vi "Subtract XY (single).vi"(8 "error in (no error)":errorcluster, 9 "y":cluster{"X-array":dbl[], "Y-array":dbl[]}, 10 "x":cluster{"X-array":dbl[], "Y-array":dbl[]}, 11 "XY-data":cluster{"X-array":dbl[], "Y-array":dbl[]}) -> (0 "error out":errorcluster, 3 "XY-data out":cluster{"X-array":dbl[], "Y-array":dbl[]} {"Y-array" format="%.2p"; "X-array" format="%.2p"})   [LabVIEW 2016, in "xy_utilities.lvlib"]
doc: "Computes the difference of the inputs.\n\n<b>x</b>'s x array is subtracted from the x array of <b>XY-data</b>\n<b>y</b>'s y array is subtracted from the y array of <b>XY-data</b>\n\nWire data to the data input to determine the polymorphic instance to use or manually select the instance."
uses:
  xy_utilities.lvlib
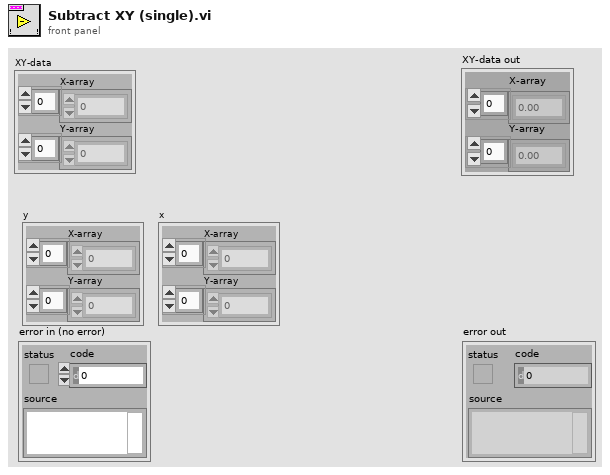
[diagram p1: front panel]
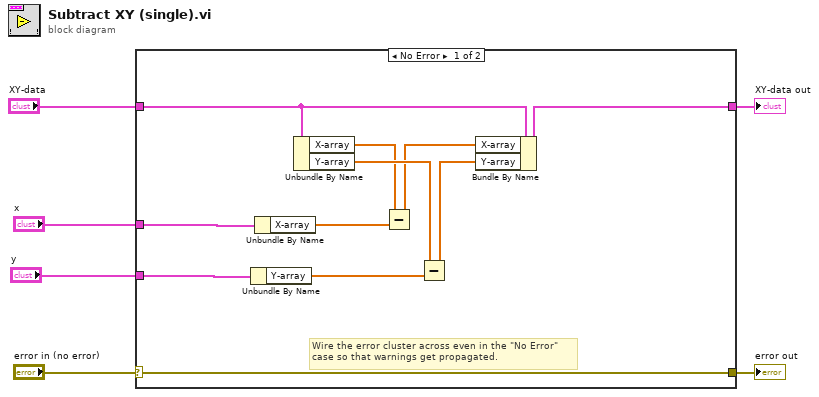
[diagram p0: block diagram]
diagram:
  n1 = case shown="No Error" "error in (no error)" {
    selector: "error in (no error)" -> [w17 w19]
    tunnel: [w17 w19] -> w5
    tunnel: "XY-data" -> [w16 w18]
    tunnel: [w15 w18] -> w3
    tunnel: "y" -> [w12 _]
    tunnel: "x" -> [w10 _]
    frame No Error {
      # "Wire the error cluster across even in the \"No Error\"\ncase so that warnings get propagated."
      n2 = Unbundle By Name(w12) -> ("Y-array"=w11:dbl[])
      n3 = Unbundle By Name(w10) -> ("X-array"=w9:dbl[])
      n4 = Unbundle By Name(w16) -> ("X-array"=w8:dbl[], "Y-array"=w14:dbl[])
      n5 = Subtract(x=w8, y=w9) -> (x-y=w7:dbl[])
      n6 = Subtract(x=w14, y=w11) -> (x-y=w13:dbl[])
      n7 = Bundle By Name(cluster=w16, "X-array"=w7, "Y-array"=w13) -> (w15:cluster{"X-array":dbl[], "Y-array":dbl[]})
    }
    frame Error {
    }
  }
  "error out" <- w5
  "XY-data out" <- w3
